vi "Match_Pat_Case_In.vi"(0 "String to match":string, 1 "String":string, 2 "offset (0)":i32) -> (3 "Before Matched string":string, 4 "Matched string":string, 5 "After  Matched string":string, 6 "offset past match":i32)   [LabVIEW 2010]
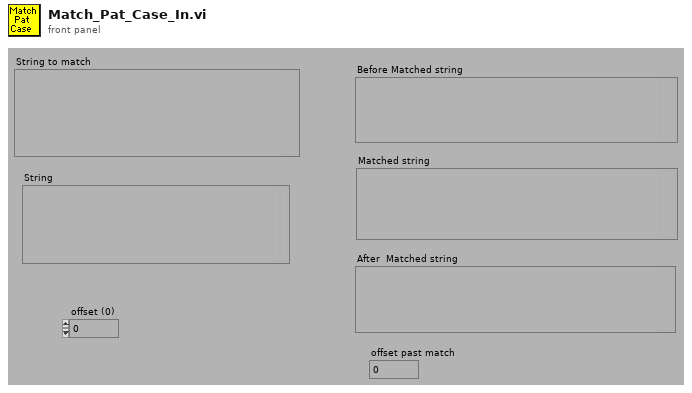
[diagram p1: front panel]
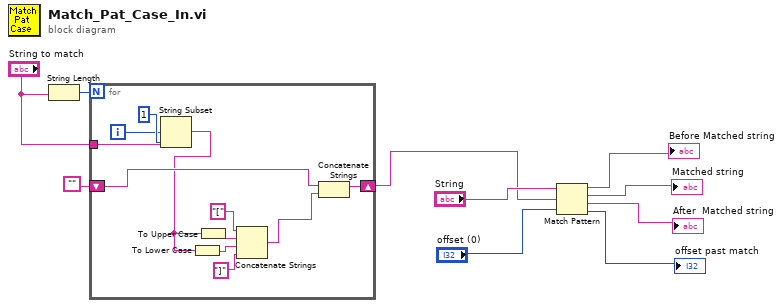
[diagram p0: block diagram]
diagram:
  n1 = String Length(string="String to match") -> (length=w3:i32)
  n2 = for {
    N: w3 -> [_]
    tunnel: "String to match" -> [w19]
    shift-right: [w17] -> w1
    shift-left: "" -> [w18]
    i -> [w20]
    n3 = String Subset(string=w19, offset (0)=w20, length (rest)=1 ("length")) -> (substring=w11:string)
    n4 = To Lower Case(string=w11) -> (all lower case string=w14:string)
    n5 = To Upper Case(1:w11) -> (0:w15:string)
    n6 = Concatenate Strings("[", w15, w14, "]" ("Substring")) -> (w16:string)
    n7 = Concatenate Strings(w18, w16) -> (w17:string)
  }
  n8 = Match Pattern(string="String", regular expression=w1, offset (0)="offset (0)") -> (before substring=→"Before Matched string":string, match substring=→"Matched string":string, after substring=→"After  Matched string":string, offset past match=→"offset past match":i32)
